vi "SSH_WriteLines.vi"(6 "search char":string="\n", 8 "error in (no error)":errorcluster, 9 "REPL":string, 10 "Buffer":string, 11 "Python in":cluster{"Python":refnum<k35>, "py file":path}) -> (0 "error out":errorcluster, 1 "Rest":string, 2 "Reply":string, 3 "Python out":cluster{"Python":refnum<k35>, "py file":path})   [LabVIEW 2020]
panel:
  out "String":string
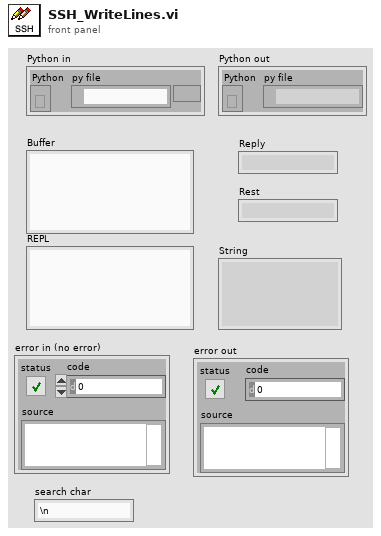
[diagram p1: front panel]
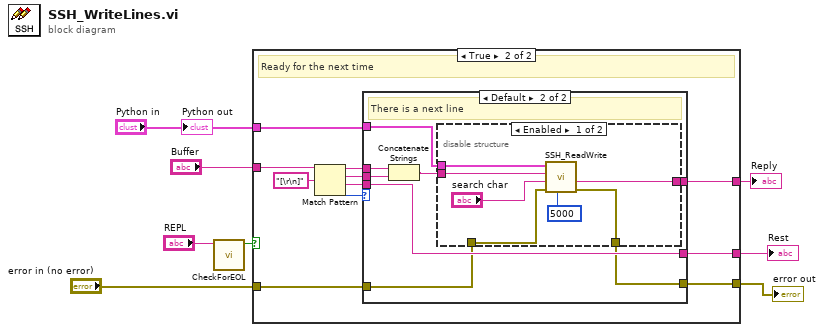
[diagram p0: block diagram]
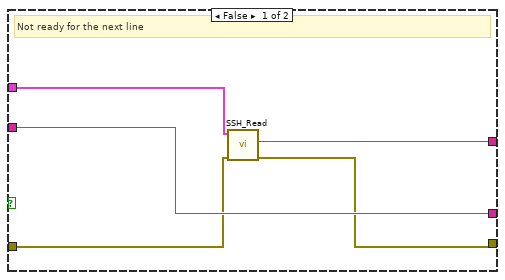
[diagram p2: hidden frame]
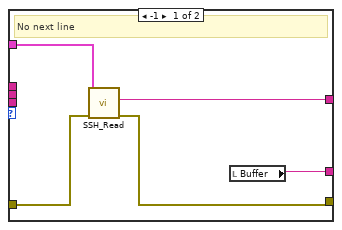
[diagram p3: hidden frame]
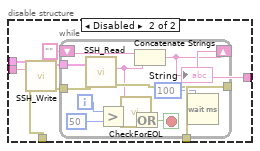
[diagram p4: hidden frame]
diagram:
  n1 = call "CheckForEOL.vi"("REPL"="REPL") -> ("Complete?"=w2:bool)  [unwired: 10 in]
  n2 = case shown="True" w2 {
    tunnel: "Buffer" -> [w13 w23]
    tunnel: [w9 w21] -> w7
    tunnel: [w13 w18] -> w1
    tunnel: "Python in" -> [w12 w16]
    tunnel: "error in (no error)" -> [w10 w15]
    tunnel: [w11 w14] -> w4
    frame False {
      # "Not ready for the next line"
      n3 = call "SSH_Read.vi"("error in (no error)"=w10, "Python in"=w12) -> ("error out"=w11:errorcluster, "Reply"=w9:string)  [unwired: 7 in, 1 out]
    }
    frame True {
      # "Ready for the next time"
      n4 = Match Pattern(string=w23, regular expression="[\r\n]") -> (before substring=w24:string, match substring=w22:string, after substring=w17:string, offset past match=w19:i32)  [unwired: 1 in]
      n5 = case shown="Default" w19 {
        tunnel: w24 -> [_ w37]
        tunnel: w22 -> [_ w35]
        tunnel: w16 -> [w28 w34]
        tunnel: [w27 w33] -> w21
        tunnel: [w29 w32] -> w18
        tunnel: w17 -> [_ w32]
        tunnel: w15 -> [w25 w31]
        tunnel: [w26 w30] -> w14
        frame -1 {
          # "No next line"
          n6 = call "SSH_Read.vi"("error in (no error)"=w25, "Python in"=w28) -> ("error out"=w26:errorcluster, "Reply"=w27:string)  [unwired: 7 in, 1 out]
          n7 = local read "Buffer"() -> (w29:string)
        }
        frame Default {
          # "There is a next line"
          n8 = Concatenate Strings(w37, w35) -> (w36:string)
          n9 = disable-structure shown="Enabled" {
            disable-tunnel: w36 -> [w43 w51]
            disable-tunnel: w34 -> [w41 w52]
            disable-tunnel: [w40 w46] -> w33
            disable-tunnel: w31 -> [w39 w49]
            disable-tunnel: [w38 w47] -> w30
            frame Enabled {
              n10 = call "SSH_ReadWrite.vi"("Timeout (ms)"=u32 5000, "error in (no error)"=w39, "Wait for"="search char", "To Send"=w43, "Python in"=w41) -> ("error out"=w38:errorcluster, "Console"=w40:string)  [unwired: 5 in]
            }
            frame Disabled {
              n11 = call "SSH_Write.vi"("error in (no error)"=w49, "Text to write"=w51, "Python in"=w52) -> ("error out"=w48:errorcluster, "Python out"=w50:cluster{"Python":refnum<k35>, "py file":path})  [unwired: 7 in]
              n12 = while {
                tunnel: w50 -> [w64]
                tunnel: w48 -> [w63]
                tunnel: [w62] -> w47
                shift-right: [w60] -> w46
                shift-left: "" -> [w61]
                i -> [w57]
                stop <- w56 stop-if-true
                n13 = call "SSH_Read.vi"("error in (no error)"=w63, "Python in"=w64) -> ("error out"=w62:errorcluster, "Reply"=w59:string)  [unwired: 7 in, 1 out]
                n14 = Greater?(x=w57, y=50) -> (0:w54:bool)
                n15 = call "CheckForEOL.vi"("REPL"=w59) -> ("Complete?"=w55:bool)  [unwired: 10 in]
                n16 = Or(x=w55, y=w54) -> (x .or. y?=w56:bool)
                n17 = Concatenate Strings(w61, w59) -> (w60:string)
                "String" <- w60
                n18 = Wait (ms)(milliseconds to wait=u32 100) -> ()  [unwired: 1 out]
              }
            }
          }
        }
      }
    }
  }
  "Reply" <- w7
  "Rest" <- w1
  "error out" <- w4
  "Python out" <- "Python in"
